vi "AutoDistancePoly.vi"   [LabVIEW 2013]
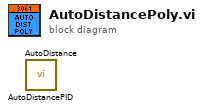
[diagram p0: block diagram]
diagram:
  n1 = call "AutoDistancePID.vi"() -> ()  [unwired: 10 in, 2 out]
  n2 = call "AutoDistance.vi"() -> ()  [unwired: 9 in, 3 out]
